vi "Read alarm XML.vi"(11 "模块名称":string) -> (3 "报警输出":string[][](array[string]))   [LabVIEW 2016, in "斯坦道氨氮.lvlib"]
uses:
  <vilib>/Utility/xml.llb/Write to XML File(string).vi
  <vilib>/Utility/xml.llb/Read From XML File(string).vi
panel:
  in  "报警常量":string[][](array[string])=[["1", "1007", "缺试剂告警", "1、建议排查管路是否异常\n2、供电情况是否正常"], ["2", "1008", "缺水样告警", "1、配水箱内无水样；\n2、配水箱到模块的管路气密性不佳；\n3、注射泵水样阀口堵塞；\n4、注射泵阀过载或丝杆无动作。"], ["3", "1009", "缺纯水告警", "1、建议排查管路是否异常\n2、供电情况是否正常"], ["4", "1010", "缺标液告警", "1、注射泵水样阀口堵塞；\n2、注射泵阀过载或丝杆无动作。"], ["5", "2007", "仪表漏液告警", "1、建议排查管路是否异常\n2、供电情况是否正常"], ["6", "1011", "标定异常告警", "1、建议排查管路是否异常\n2、供电情况是否正常"], ["7", "4", "超量程告警", "1、建议排查管路是否异常\n2、供电情况是否正常"], ["8", "2008", "加热告警", "检查温度传感器、检查加热片是否损坏或脱落、检查加热模块与电路板接线是否正常、检查固件是否匹配"], ["9", "1051", "低试剂预警", "1、建议排查管路是否异常\n2、供电情况是否正常"], ["10", "1", "超上限告警", "1、建议排查管路是否异常\n2、供电情况是否正常"], ["11", "2", "超下限告警", "1、建议排查管路是否异常\n2、供电情况是否正常"], ["12", "1012", "其他告警", "1、建议排查管路是否异常\n2、供电情况是否正常"], ["13", "1028", "滴定异常告警", "1、建议排查管路是否异常\n2、供电情况是否正常"], ["14", "1069", "电极异常告警", "1、建议排查管路是否异常\n2、供电情况是否正常"], ["15", "3", "量程切换告警", "1、建议排查管路是否异常\n2、供电情况是否正常"], ["16", "1070", "参数设置告警", "1、建议排查管路是否异常\n2、供电情况是否正常"], ["17", "1071", "pH电极电位异常", "1、建议排查管路是否异常\n2、供电情况是否正常"], ["18", "1072", "电导率电极异常", "1、建议排查管路是否异常\n2、供电情况是否正常"], ["19", "1073", "浊度光度异常", "1、建议排查管路是否异常\n2、供电情况是否正常"], ["20", "1074", "溶解氧电极异常", "1、建议排查管路是否异常\n2、供电情况是否正常"], ["21", "1075", "溶解氧光强异常", "1、建议排查管路是否异常\n2、供电情况是否正常"], ["22", "1076", "温度异常告警", "1、建议排查管路是否异常\n2、供电情况是否正常"], ["23", "1077", "pH异常告警", "1、建议排查管路是否异常\n2、供电情况是否正常"], ["24", "1078", "溶解氧异常告警", "1、建议排查管路是否异常\n2、供电情况是否正常"], ["25", "1079", "电导率异常告警", "1、建议排查管路是否异常\n2、供电情况是否正常"], ["26", "1080", "浊度异常告警", "1、建议排查管路是否异常\n2、供电情况是否正常"], ["27", "1081", "叶绿素a异常告警", "1、建议排查管路是否异常\n2、供电情况是否正常"], ["28", "1082", "藻密度异常告警", "1、建议排查管路是否异常\n2、供电情况是否正常"], ["29", "1083", "蓝绿藻异常告警", "1、建议排查管路是否异常\n2、供电情况是否正常"], ["30", "1084", "ORP异常告警", "1、建议排查管路是否异常\n2、供电情况是否正常"], ["31", "1085", "氨氮异常告警", "1、建议排查管路是否异常\n2、供电情况是否正常"], ["32", "1086", "清洁刷异常告警", "1、建议排查管路是否异常\n2、供电情况是否正常"], ["33", "1087", "SD卡异常告警", "1、建议排查管路是否异常\n2、供电情况是否正常"], ["34", "1088", "蓝牙异常告警", "1、建议排查管路是否异常\n2、供电情况是否正常"], ["35", "1089", "WIFI异常告警", "1、建议排查管路是否异常\n2、供电情况是否正常"], ["36", "1013", "缺流程告警", "流程未写入、芯片异常，未存储"], ["37", "1014", "芯片存储异常告警", "固件异常"], ["38", "1015", "缺公式告警", "公式未写入、芯片异常，未存储"], ["40", "6", "光值过低告警", "1、检查比色皿是否污染严重；\n2、检查水体浊度是否过高。"], ["41", "5", "光值过高告警", "检查光强是否漂移"], ["42", "1017", "温度探头接线异常告警", "1、建议排查管路是否异常\n2、供电情况是否正常"], ["43", "1018", "温度探头未嵌入凹槽或消解模", "1、建议排查管路是否异常\n2、供电情况是否正常"], ["44", "1019", "温度探头功率过大告警", "1、建议排查管路是否异常\n2、供电情况是否正常"], ["61", "1008", "缺水样告警", "1、建议排查管路是否异常\n2、供电情况是否正常"], ["62", "1010", "缺标样告警", "1、建议排查管路是否异常\n2、供电情况是否正常"], ["63", "1046", "缺零点核查样告警", "1、建议排查管路是否异常\n2、供电情况是否正常"], ["64", "1047", "缺跨度核查样告警", "1、建议排查管路是否异常\n2、供电情况是否正常"], ["65", "1048", "缺空白样告警", "1、建议排查管路是否异常\n2、供电情况是否正常"], ["66", "1049", "缺平行样告警", "1、建议排查管路是否异常\n2、供电情况是否正常"], ["67", "1050", "缺加标样告警", "1、建议排查管路是否异常\n2、供电情况是否正常"], ["70", "1051", "缺试剂A", "1、建议排查管路是否异常\n2、供电情况是否正常"], ["71", "1052", "缺试剂B", "1、建议排查管路是否异常\n2、供电情况是否正常"], ["81", "1053", "水样余量过低，请及时维护", "1、建议排查管路是否异常\n2、供电情况是否正常"], ["82", "1054", "标液余量过低，请及时维护", "1、建议排查管路是否异常\n2、供电情况是否正常"], ["83", "1055", "零点样余量过低，请及时维护", "1、建议排查管路是否异常\n2、供电情况是否正常"], ["84", "1056", "跨度样余量过低，请及时维护", "1、建议排查管路是否异常\n2、供电情况是否正常"], ["85", "1057", "空白样余量过低，请及时维护", "1、建议排查管路是否异常\n2、供电情况是否正常"], ["86", "1058", "平行样余量过低，请及时维护", "1、建议排查管路是否异常\n2、供电情况是否正常"], ["87", "1059", "加标样余量过低，请及时维护", "1、建议排查管路是否异常\n2、供电情况是否正常"], ["90", "1060", "试剂A余量过低，请及时维护", "1、建议排查管路是否异常\n2、供电情况是否正常"], ["91", "1061", "试剂B余量过低，请及时维护", "1、建议排查管路是否异常\n2、供电情况是否正常"], ["99", "1023", "注射泵配置异常告警", "代码99：检查流程是否错误，查询注射泵配置信息是否不匹配"], ["103", "1020", "注射泵供电异常告警", "代码103：注射泵未初始化，检查电压是否正常"], ["105", "1021", "注射泵丝杆过载告警", "代码105：检查丝杆是否生锈、检查注射器阻力是否正常、检查注射泵自检是否正常"], ["106", "1022", "注射泵阀头切换过载告警", "代码106：检查阀口是否堵塞、检查多通阀转子接触面是否黏结"], ["250", "1062", "请注意查看溶液或试剂余量并", "1、建议排查管路是否异常\n2、供电情况是否正常"], ["253", "1063", "旋转阀通讯异常告警", "1、建议排查管路是否异常\n2、供电情况是否正常"], ["254", "1025", "光谱仪通讯异常告警", "1、建议排查管路是否异常\n2、供电情况是否正常"], ["255", "1024", "注射泵通讯异常告警", "代码255：检查注射泵与电路板通讯是否正常"], ["500", "1090", "试剂不足", "试剂不足，请及时补充试剂"], ["501", "1091", "试剂余量检测异常", "请查询固件流程是否匹配，试剂是否有倒灌现象"]]
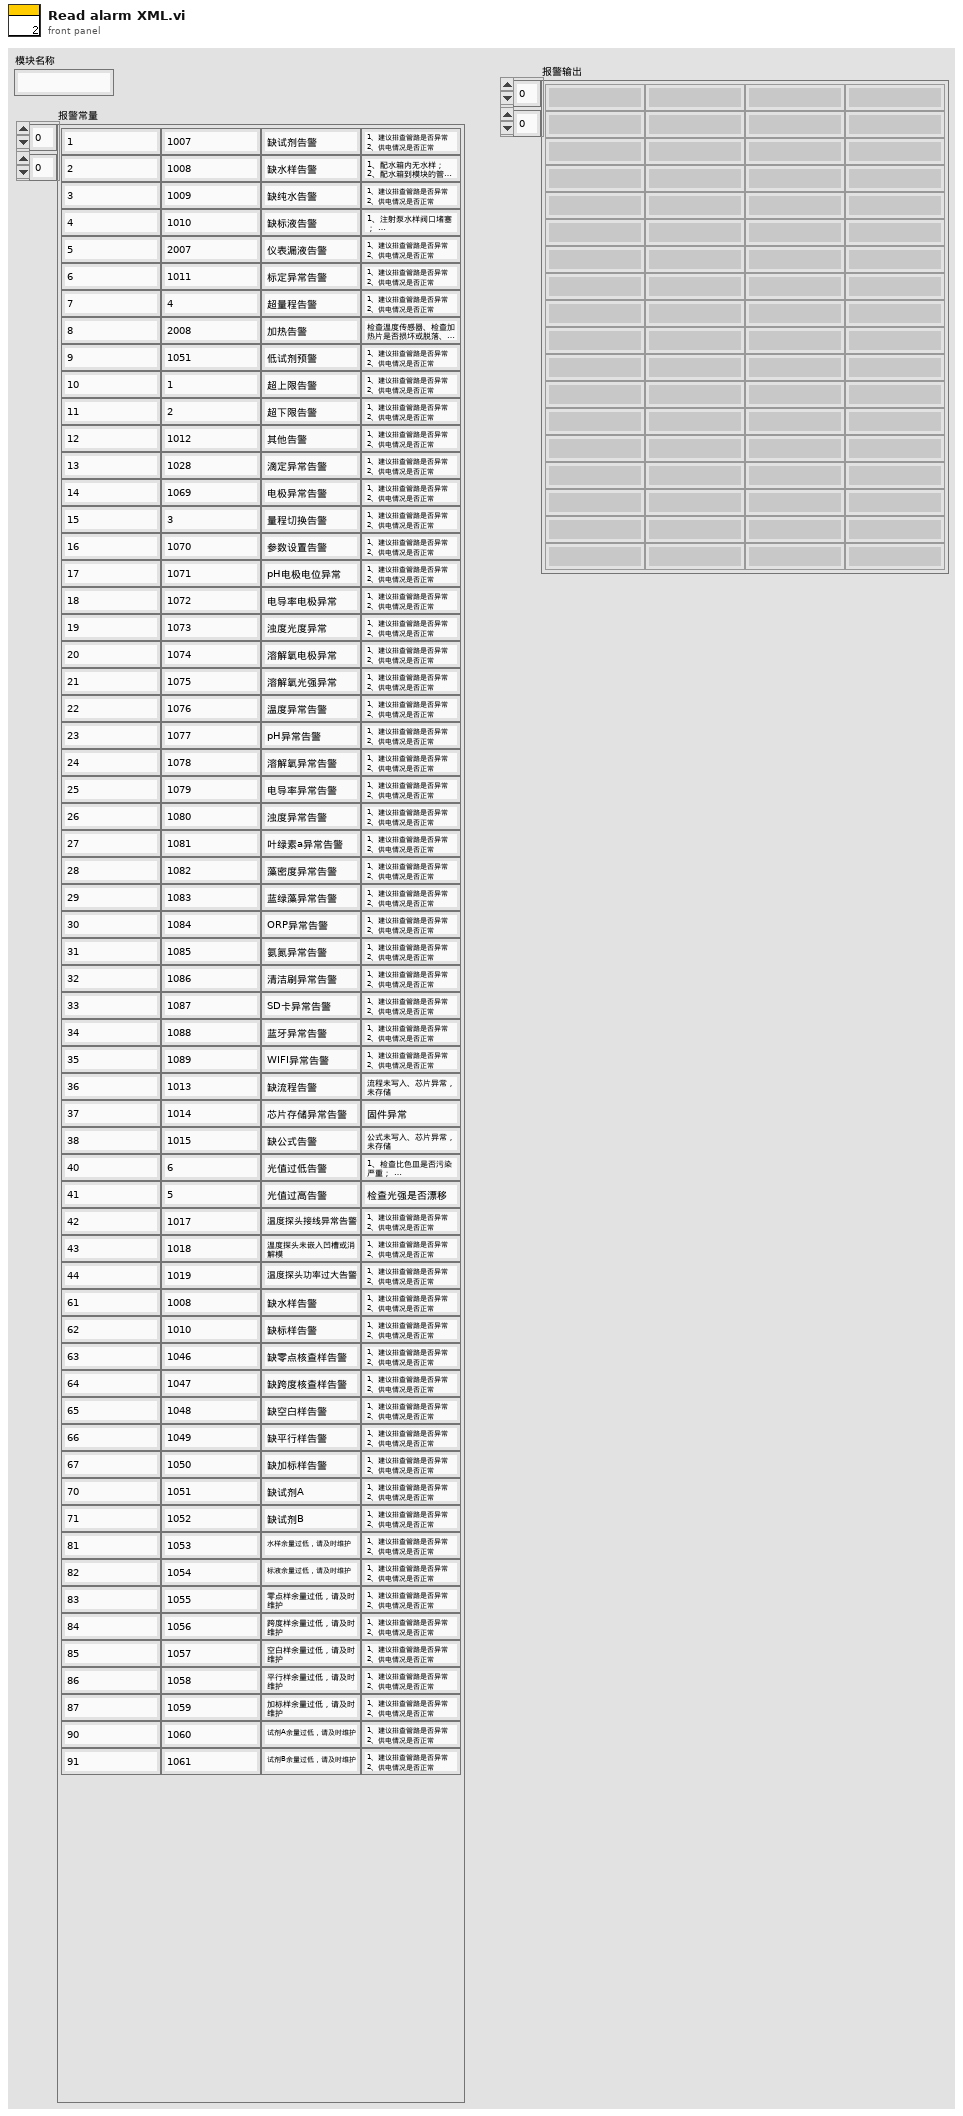
[diagram p1: front panel]
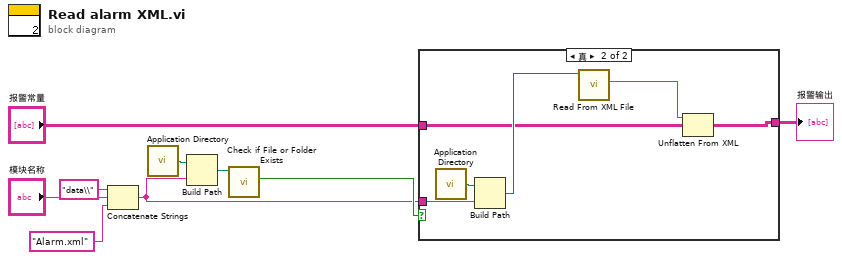
[diagram p0: block diagram]
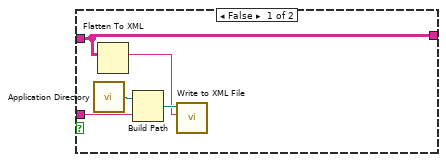
[diagram p2: hidden frame]
diagram:
  n1 = Concatenate Strings("data\\" ("字符串"), "模块名称", "Alarm.xml" ("名称或相对路径")) -> (w6:string)
  n2 = call <vilib>:"Application Directory.vi"() -> ("Application Directory"=w4:path)
  n3 = Build Path(base path=w4, name or relative path=w6) -> (appended path=w5:path)
  n4 = call <vilib>:"Check if File or Folder Exists.vi"("path"=w5) -> ("file or folder exists?"=w7:bool)  [unwired: 8 in, 2 out]
  n5 = case shown="真" w7 {
    tunnel: [w10 w17] -> w8
    tunnel: w6 -> [w11 w16]
    tunnel: "报警常量" -> [w10 w15]
    frame False {
      n6 = call <vilib>:"Application Directory.vi"() -> ("Application Directory"=w13:path)
      n7 = Flatten To XML(anything=w10) -> (xml string=w12:string)
      n8 = Build Path(base path=w13, name or relative path=w11) -> (appended path=w14:path)
      n9 = call-poly <vilib>:"Write to XML File.vi"("XML Input"=w12, "XML File Path"=w14) -> ()  [unwired: 7 in, 3 out]
    }
    frame True {
      n10 = call <vilib>:"Application Directory.vi"() -> ("Application Directory"=w19:path)
      n11 = Build Path(base path=w19, name or relative path=w16) -> (appended path=w18:path)
      n12 = call-poly <vilib>:"Read From XML File.vi"("XML File Path"=w18) -> ("XML Elements"=w20:string)  [unwired: 8 in, 2 out]
      n13 = Unflatten From XML(xml string=w20, type=w15) -> (value=w17:string[][])  [unwired: 1 in, 1 out]
    }
  }
  "报警输出" <- w8
